vi "Lorentzian complex model.vi"() -> ()   [LabVIEW 2016]
uses:
  <vilib>/Analysis/3filter.llb/Filter Passband Type.ctl
  <vilib>/Analysis/3filter.llb/Butterworth Filter (CDB).vi
  <vilib>/Analysis/NI_AAL_SigProc.lvlib
  <vilib>/Analysis/NI_AALBase.lvlib
panel:
  in  "Low pass distortion":dbl
  out "Gama guess":dbl
  out "2nd Derivatives":dbl[](array[numeric])
  out "Amplitudes":dbl[](array[numeric])
  out "Locations":dbl[](array[numeric])
  out "Waveform Graph 2":dbl[](graph)
  out "standard deviation":dbl format="%0.2f"
  out "Circle plot":cluster{dbl[], dbl[]}[](graph)
  in  "phase":dbl
  in  "Amplitude":dbl=50.0
  in  "Range":i32=100
  in  "Gamma":dbl=10.0
  in  "F0":dbl=50.0
  out "Waveform Graph":dbl[][](graph)
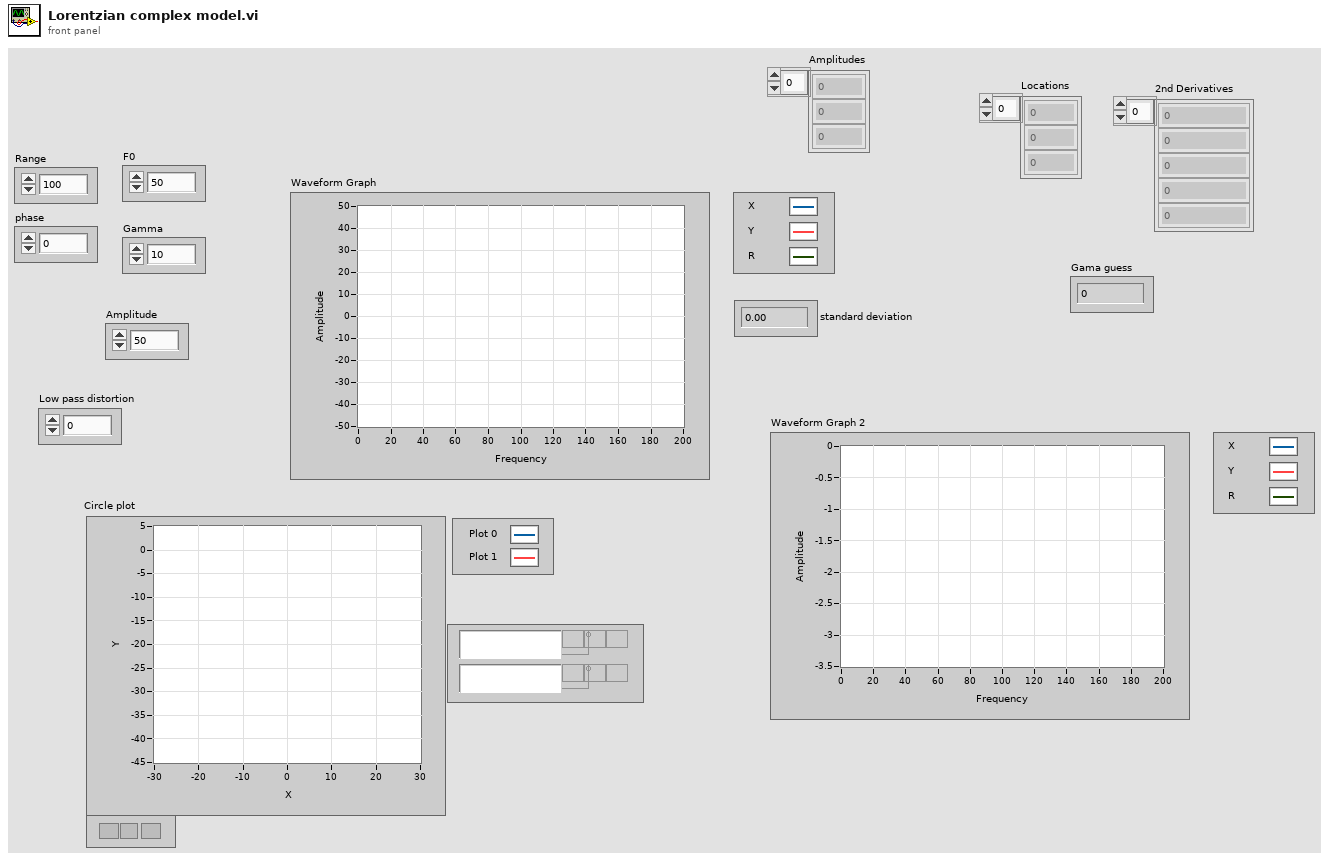
[diagram p1: front panel]
types:
  T1 = typedef "NI_AALBase.lvlib/Filter Passband Type.ctl" = enum32{"Lowpass", "Highpass", "Bandpass", "Bandstop"}
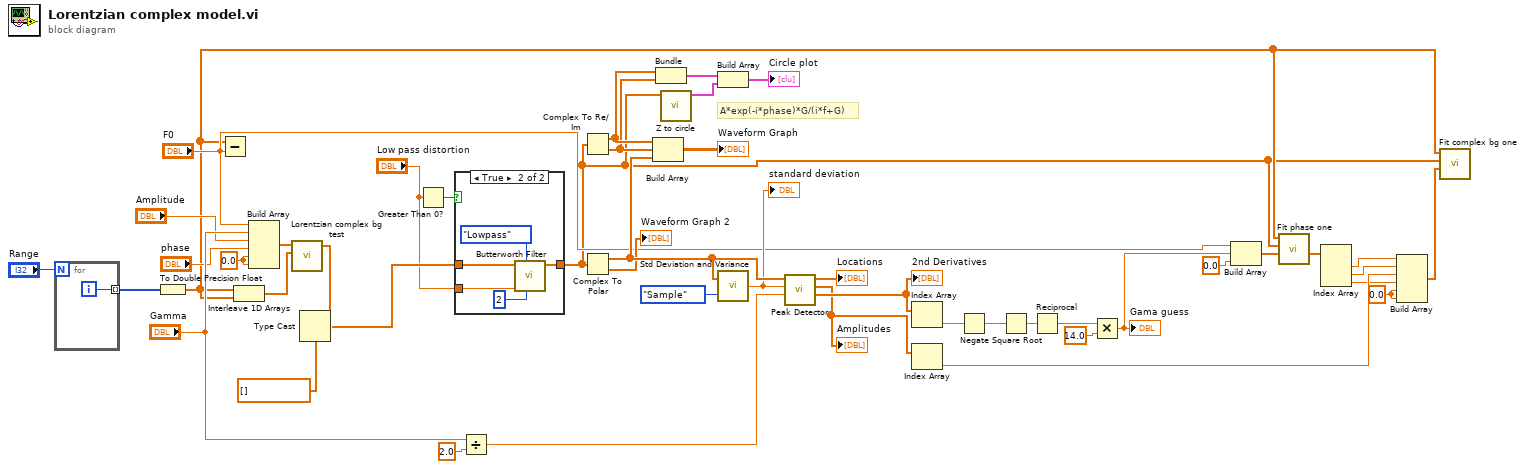
[diagram p0: block diagram]
diagram:
  w10 = 0.0
  w17 = 0.0 ("element")
  # "A*exp(-i*phase)*G/(i*f+G)"
  n1 = for {
    N: "Range" -> [_]
    tunnel: [w47] -> w25 mode=indexing
    i -> [w47]
  }
  n2 = To Double Precision Float(number=w25) -> (double precision float=w8:dbl[])
  n3 = Subtract(x=w8, y="F0") -> ()  [unwired: 1 out]
  n4 = Interleave 1D Arrays(w8, w8) -> (w7:dbl[])
  n5 = Build Array("F0", "Gamma", "Amplitude", "phase", w10, w10) -> (w9:dbl[])
  n6 = call "Lorentzian complex bg test.vi"("X"=w7, "a"=w9) -> ("f(X,a)"=w5:dbl[])  [unwired: 2 in, 2 out]
  n7 = Type Cast(type=cdb[] [] ("x*y"), x=w5) -> (*(type *) &x=w3:cdb[])
  n8 = Greater Than 0?(x="Low pass distortion") -> (x > 0?=w4:bool)
  n9 = case shown="True" w4 {
    tunnel: w3 -> [w48 w53]
    tunnel: [w48 w52] -> w2
    tunnel: "Low pass distortion" -> [_ w50]
    frame False {
    }
    frame True {
      n10 = call-poly <vilib>:"Butterworth Filter.vi"("order"=2, "filter type"=Filter_Passband_Type."Lowpass", "low cutoff freq: fl"=w50, "X"=w53) -> ("Filtered X"=w52:cdb[])  [unwired: 4 in, 1 out]
    }
  }
  n11 = Divide(x="Gamma", y=2.0) -> (x/y=w27:dbl)
  n12 = Complex To Re/Im(x + iy=w2) -> (x=w44:dbl[], y=w43:dbl[])
  n13 = Complex To Polar(r * e^(i*theta)=w2) -> (r=w41:dbl[], theta=→"Waveform Graph 2":dbl[])
  n14 = Build Array(w44, w43, w41) -> (→"Waveform Graph":dbl[][])
  n15 = Bundle(w44, w43) -> (w42:cluster{dbl[], dbl[]})  [unwired: 1 in]
  n16 = call "Z to circle.vi"("Z"=w2) -> ("plot"=w15:cluster{"Array":dbl[], "Array":dbl[]})  [unwired: 6 in, 4 out]
  n17 = Build Array(w42, w15) -> (→"Circle plot":cluster{"Array":dbl[], "Array":dbl[]}[])
  n18 = call <vilib>:"Std Deviation and Variance.vi"("X"=w41, "Weighting (Sample)"=enum16{"Sample", "Population"}."Sample") -> ("standard deviation"=w39:dbl)  [unwired: 2 out]
  "standard deviation" <- w39
  n19 = call <vilib>:"Peak Detector.vi"("width"=w27, "threshold"=w39, "X"=w41) -> ("2nd Derivatives"=w33:dbl[], "Amplitudes"=w20:dbl[], "Locations"=→"Locations":dbl[])  [unwired: 4 in, 2 out]
  "Amplitudes" <- w20
  "2nd Derivatives" <- w33
  n20 = Index Array(array=w33) -> (element=w32:dbl)  [unwired: 1 in]
  n21 = Index Array(array=w20) -> (element=w19:dbl)  [unwired: 1 in]
  n22 = Negate(x=w32) -> (-x=w31:dbl)
  n23 = Square Root(x=w31) -> (sqrt(x)=w30:dbl)
  n24 = Reciprocal(x=w30) -> (1/x=w29:dbl)
  n25 = Multiply(x=w29, y=14.0) -> (x*y=w26:dbl)
  "Gama guess" <- w26
  n26 = Build Array("F0", w26, 0.0 ("element")) -> (w35:dbl[])
  n27 = call "Fit phase one.vi"("Initial parameters"=w35, "Z"=w2, "X"=w8) -> ("best fit parameters"=w23:dbl[])  [unwired: 8 in]
  n28 = Index Array(array=w23) -> (element #1=w22:dbl, element #2=w21:dbl, element #3=w18:dbl)  [unwired: 3 in]
  n29 = Build Array(w22, w21, w19, w18, w17, w17) -> (w24:dbl[])
  n30 = call "Fit complex bg one.vi"("Initial parameters"=w24, "Z"=w2, "X"=w8) -> ()  [unwired: 9 in]
